vi "GetID.vi"(8 "error in (no error)":errorcluster, 11 "reference in":refnum<class "Oven.lvclass">) -> (0 "error out":errorcluster, 2 "Id String":string, 3 "reference in":refnum<class "Oven.lvclass">)   [LabVIEW 2020, in "Oven.lvclass"]
uses:
  Oven.lvclass
  Equipment_class/Equipment.lvclass
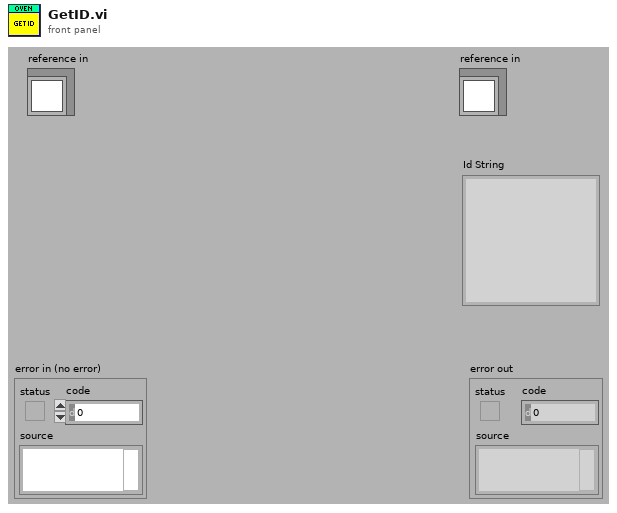
[diagram p1: front panel]
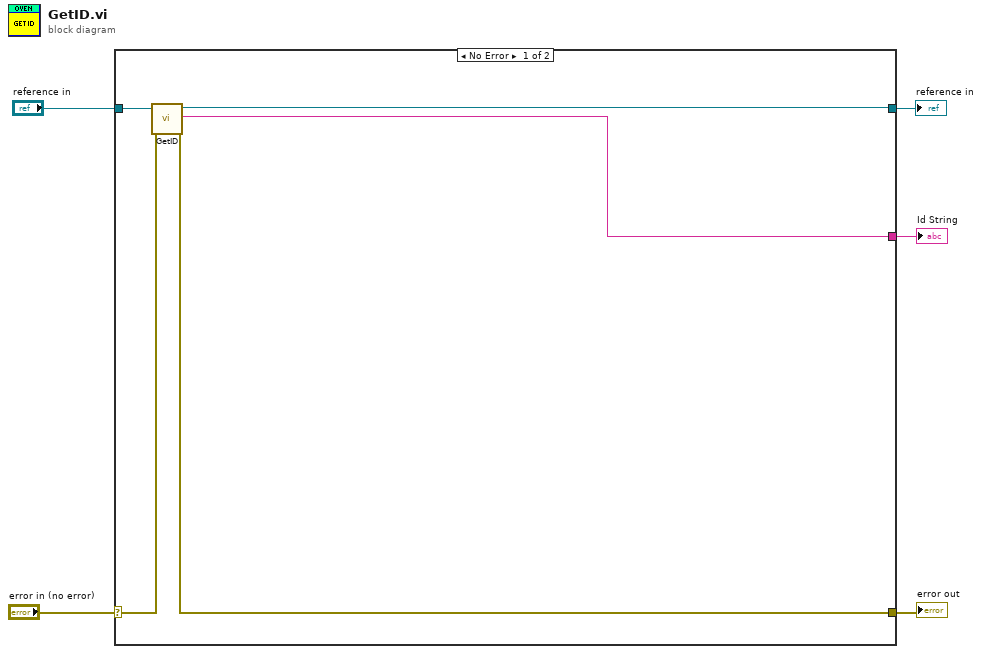
[diagram p0: block diagram]
diagram:
  n1 = case shown="No Error" "error in (no error)" {
    selector: "error in (no error)" -> [w9 w12]
    tunnel: [w8 w12] -> w4
    tunnel: [w7 w11] -> w2
    tunnel: "reference in" -> [w10 w11]
    tunnel: [w6 _] -> w1
    frame No Error {
      n2 = call-parent "GetID.vi"("error in (no error)"=w9, "reference in"=w10) -> ("error out"=w8:errorcluster, "Id String"=w6:string, "reference out"=w7:refnum<class "Oven.lvclass">)  [unwired: 7 in]
    }
    frame Error {
    }
  }
  "error out" <- w4
  "reference in" <- w2
  "Id String" <- w1
